vi "Plugin Pre-Build Action.vi"(6 "Top Level/Always Included VIs":path[](array[path]), 7 "Main Destination Path":path, 9 "Target Name":string, 10 "Build Specification Name":string, 11 "Project Path":path) -> (0 "error out":errorcluster)   [LabVIEW 2021, in "CIF Build Actions.lvlib"]
uses:
  CIF Build Actions.lvlib
  <vilib>/AppBuilder/AB_API/common/AB_API Build Object Selector.ctl
  <vilib>/AppBuilder/AB_API/PPL/NI_AB_API_PPL.lvclass
  CIFCore/Common/Typedef/Errors.ctl
  CIFCore/Common/Utilities/Append Error Location.vi
  <vilib>/AppBuilder/AB_API/Build/NI_AB_API_Build.lvclass
  CIFCore/Common/CIFCoreCommon.lvlib
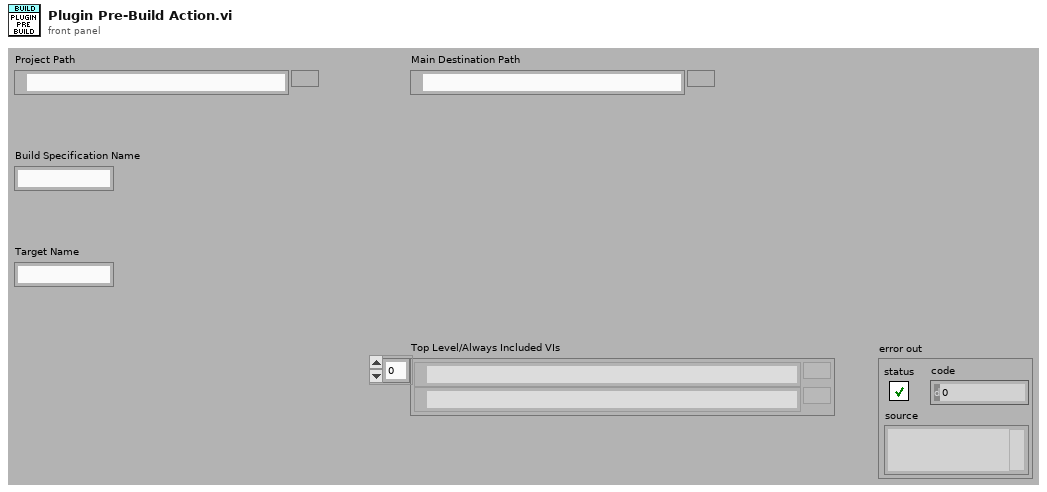
[diagram p1: front panel]
types:
  T1 = cluster{"Major":u16, "Minor":u16, "Fix":u16, "Build":u16}
  T2 = typedef "AB_API Build Object Selector.ctl" = enum16{"Source Distribution", "Deployable Source Distribution", "DLL", "EXE", "Packed Library", "Deployable Packed Library", "RT EXE", ".NET Interop Assembly"}
  T3 = typedef "CIFCoreCommon.lvlib/Errors.ctl" = enum16{"Invalid Clock ID", "Long Sleep", "gRPC Server Not Found", "Config Parse", "Timestamp Wrap", "Delayed Execution", "Duplicate Channel", "Missing Channel", "Incorrect Type", "Flatten Error", "Unflatten Data", "Unique Name", "Plugin Not Found", "Plugin Type Not Found", "Plugin Version Not Found", "Manager Not Found", "Numerical Issue", "Time Jump", "Clock ID Match", "Channel Length", "Plugin Connection", "gRPC Server Connection", "PPL Name Match", "Build"}
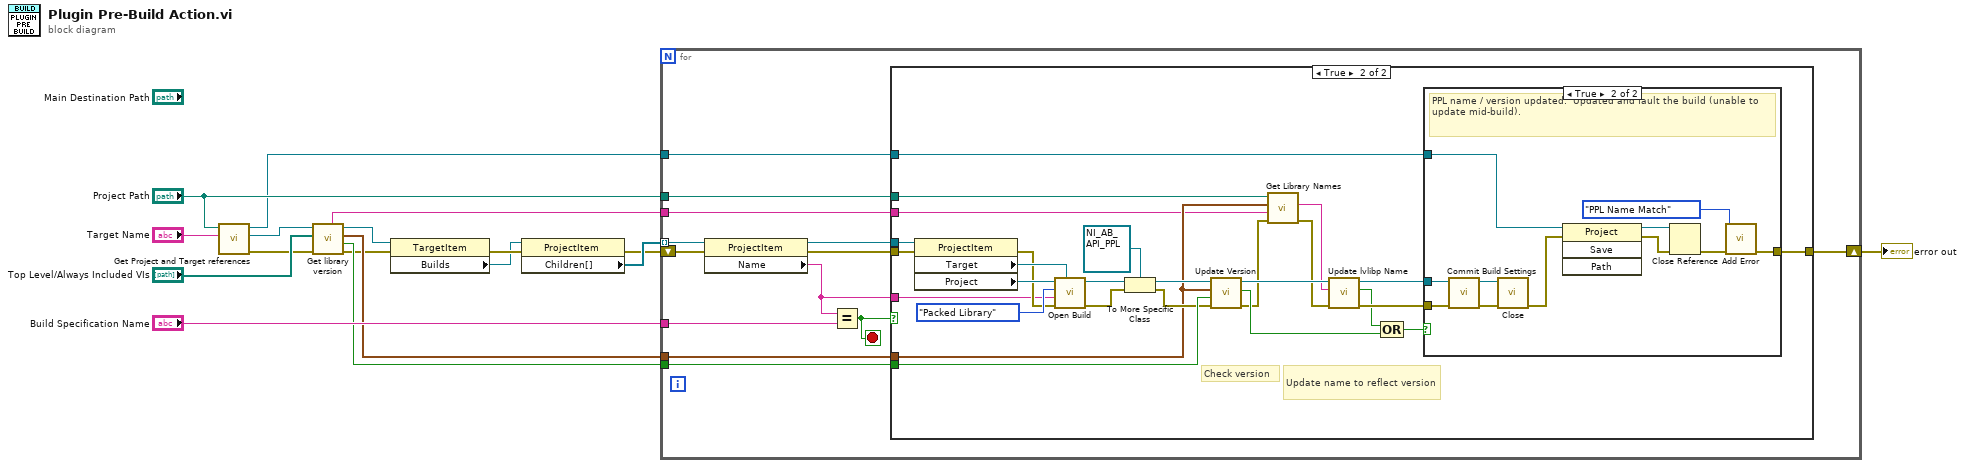
[diagram p0: block diagram]
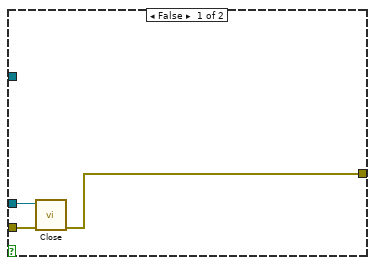
[diagram p3: hidden frame]
diagram:
  n1 = call "Get Project and Target references.vi"("Target Name"="Target Name", "Project Path"="Project Path") -> ("error out"=w6:errorcluster, "Target refnum"=w8:refnum<vi>, "Project refnum"=w2:refnum<vi>)  [unwired: 7 in]
  n2 = call "Get library version.vi"("error in (no error)"=w6, "Top Level/Always Included VIs"="Top Level/Always Included VIs", "Target reference in"=w8) -> ("error out"=w3:errorcluster, "Library Found"=w9:bool, "Version"=w10:T1, "Target reference out"=w7:refnum<vi>, "found library name"=w1:string)  [unwired: 4 in]
  n3 = property class="TargetItem"(reference=w7, error in=w3) -> (error out=w16:errorcluster, "Builds"=w15:refnum<vi>)  [unwired: 1 out]
  n4 = property class="ProjectItem"(reference=w15, error in=w16) -> (error out=w5:errorcluster, "Children[]"=w17:refnum<vi>[])  [unwired: 1 out]
  n5 = for {
    tunnel: w17 -> [w29] mode=indexing
    tunnel: w10 -> [w30]
    tunnel: w9 -> [w23]
    shift-right: [w25] -> w13
    shift-left: w5 -> [w26]
    tunnel: w2 -> [w21]
    tunnel: "Build Specification Name" -> [w20]
    tunnel: "Project Path" -> [w19]
    tunnel: w1 -> [w18]
    stop <- w22 stop-if-true
    n6 = property class="ProjectItem"(reference=w29, error in=w26) -> (reference out=w28:refnum<vi>, error out=w27:errorcluster, "Name"=w24:string)
    n7 = Equal?(x=w24, y=w20) -> (x = y?=w22:bool)
    n8 = case shown="True" w22 {
      tunnel: w30 -> [_ w36]
      tunnel: w28 -> [_ w51]
      tunnel: w27 -> [w31 w50]
      tunnel: [w31 w49] -> w25
      tunnel: w24 -> [_ w47]
      tunnel: w23 -> [_ w48]
      tunnel: w21 -> [_ w46]
      tunnel: w19 -> [_ w37]
      tunnel: w18 -> [_ w33]
      frame False {
      }
      frame True {
        # "Update name to reflect version"
        # "Check version"
        n9 = property class="ProjectItem"(reference=w51, error in=w50) -> (error out=w52:errorcluster, "Target"=w58:refnum<vi>, "Project"=w57:refnum<vi>)  [unwired: 1 out]
        n10 = call <vilib>:"Open Build.vi"("TargetItem Refnum"=w58, "error in (no error)"=w52, "Build specification name"=w47, "Build object selector"=AB_API_Build_Object_Selector."Packed Library", "Project Refnum"=w57) -> ("error out"=w53:errorcluster, "NI_AB_API_Build out"=w55:refnum<class "NI_AB_API_Build.lvclass">)  [unwired: 5 in]
        n11 = To More Specific Class(target class=refnum<class "NI_AB_API_PPL.lvclass"> refnum ("PPL out"), reference=w55, error in=w53) -> (specific class reference=w45:refnum<class "NI_AB_API_PPL.lvclass">, error out=w44:errorcluster)
        n12 = call "Update Version.vi"("error in (no error)"=w44, "Valid"=w48, "Library Version"=w36, "NI_AB_API_PPL in"=w45) -> ("error out"=w35:errorcluster, "Updated"=w39:bool, "NI_AB_API_PPL out"=w43:refnum<class "NI_AB_API_PPL.lvclass">)  [unwired: 5 in]
        n13 = call "Get Library Names.vi"("error in (no error)"=w35, "Override Name"=w33, "Version"=w36, "Project Path"=w37) -> ("error out"=w34:errorcluster, "Versioned Library"=w32:string)  [unwired: 4 in, 2 out]
        n14 = call "Update lvlibp Name.vi"("error in (no error)"=w34, "lvlibp name"=w32, "NI_AB_API_PPL in"=w43) -> ("error out"=w42:errorcluster, "Updated"=w40:bool, "NI_AB_API_PPL out"=w41:refnum<class "NI_AB_API_PPL.lvclass">)  [unwired: 6 in]
        n15 = Compound Arithmetic op=OR(w40, w39) -> (w38:bool)
        n16 = case shown="True" w38 {
          tunnel: [w61 w66] -> w49
          tunnel: w46 -> [_ w62]
          tunnel: w42 -> [w59 w64]
          tunnel: w41 -> [w60 w63]
          frame False {
            n17 = call-dynamic "Close.vi"("error in (no error)"=w59, "DLL in"=w60) -> ("error out"=w61:errorcluster)  [unwired: 9 in]
          }
          frame True {
            # "PPL name / version updated.  Updated and fault the build (unable to update mid-build)."
            n18 = call-dynamic "Commit Build Settings.vi"("error in (no error)"=w64, "PPL in"=w63) -> ("error out"=w71:errorcluster, "PPL out"=w72:refnum<class "NI_AB_API_PPL.lvclass">)  [unwired: 8 in]
            n19 = call-dynamic "Close.vi"("error in (no error)"=w71, "DLL in"=w72) -> ("error out"=w68:errorcluster)  [unwired: 9 in]
            n20 = invoke class="Project" method="Save"(reference=w62, error in=w68) -> (reference out=w69:refnum<vi>, error out=w70:errorcluster)  [unwired: 2 in, 2 out]
            n21 = Close Reference(reference=w69, error in (no error)=w70) -> (error out=w67:errorcluster)
            n22 = call "Add Error.vi"("error in (no error)"=w67, "Error"=Errors."PPL Name Match") -> ("error out"=w66:errorcluster)  [unwired: 9 in]
          }
        }
      }
    }
  }
  "error out" <- w13
